vi "Untitled 1.vi"() -> ()   [LabVIEW 2018]
uses:
  <vilib>/addons/control/pid/pid.llb/PID (DBL).vi
  <vilib>/addons/control/pid/NI_PID_pid.lvlib
panel:
  in  "rand multiplier":dbl
  in  "PID gains":T1={"proportional gain (Kc)"=1.0, "integral time (Ti, min)"=0.01, "derivative time (Td, min)"=0.0} {"derivative time (Td, min)" format="%.3g"; "integral time (Ti, min)" format="%.3g"; "proportional gain (Kc)" format="%.3g"}
  out "output":cluster{"output":dbl, "dt out (s)":dbl}(graph)
  in  "setpoint":dbl format="%.2f"
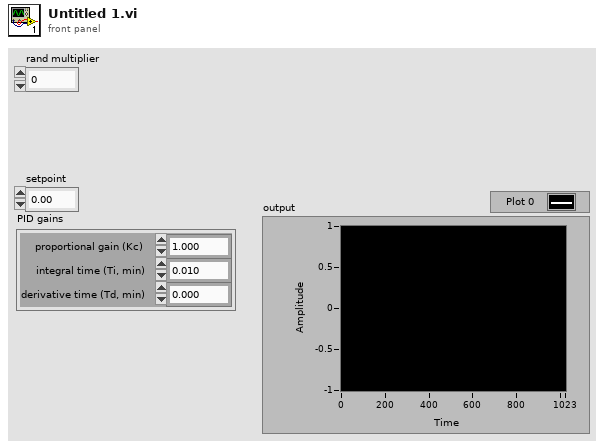
[diagram p1: front panel]
types:
  T1 = cluster{"proportional gain (Kc)":dbl, "integral time (Ti, min)":dbl, "derivative time (Td, min)":dbl}
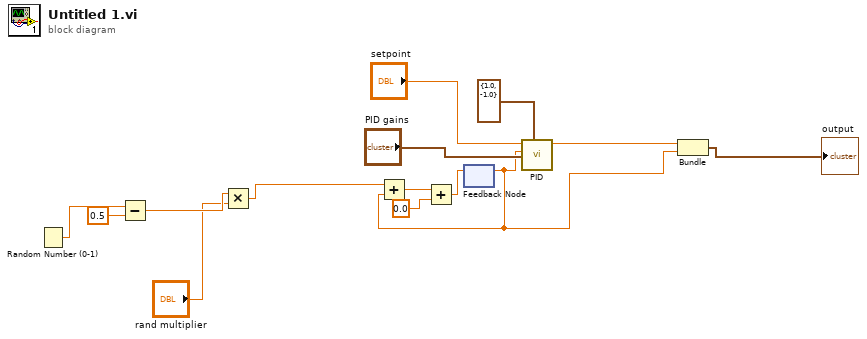
[diagram p0: block diagram]
diagram:
  n1 = Random Number (0-1)() -> (number: 0 to 1=w5:dbl)
  n2 = Subtract(x=w5, y=0.5) -> (x-y=w3:dbl)
  n3 = Multiply(x=w3, y="rand multiplier") -> (x*y=w1:dbl)
  n4 = feedback #1() -> (w6:dbl)  [unwired: 1 in]
  n5 = Add(x=w1, y=w6) -> (x+y=w12:dbl)
  n6 = Add(x=w12, y=0.0) -> (x+y=w10:dbl)
  n7 = feedback-in #1(w10) -> ()
  n8 = call-poly <vilib>:"PID.vi"("output range"=cluster{"output high":dbl, "output low":dbl} {"output high"=1.0, "output low"=-1.0}, "PID gains"="PID gains", "process variable"=w6, "setpoint"="setpoint") -> ("output"=w8:dbl)  [unwired: 6 in, 1 out]
  n9 = Bundle("output"=w8, w6) -> (→"output":cluster{"output":dbl, dbl})  [unwired: 1 in]
